vi "Read Voffset.vi"(8 "error in (no error)":errorcluster, 11 "Change Speaker Vparams in":refnum<class "Change Speaker Vparams.lvclass">) -> (0 "error out":errorcluster, 2 "Voffset":dbl, 3 "Change Speaker Vparams out":refnum<class "Change Speaker Vparams.lvclass">)   [LabVIEW 2014, in "ePAS Library.lvlib" / "Change Speaker Vparams.lvclass"]
uses:
  Change Speaker Vparams.lvclass
  Change Speaker Vparams.lvclass/Change Speaker Vparams.ctl
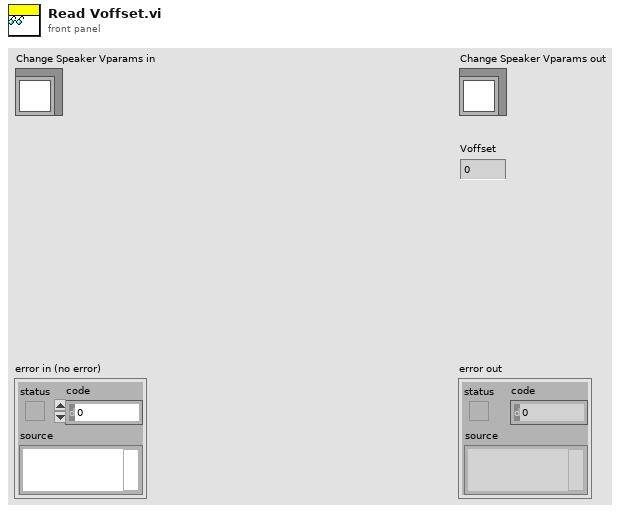
[diagram p1: front panel]
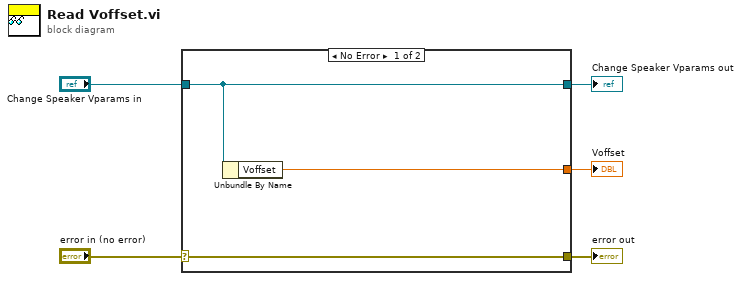
[diagram p0: block diagram]
diagram:
  n1 = case shown="No Error" "error in (no error)" {
    selector: "error in (no error)" -> [w8 w9]
    tunnel: [w8 w9] -> w4
    tunnel: [w7 w10] -> w2
    tunnel: "Change Speaker Vparams in" -> [w7 w10]
    tunnel: [w6 _] -> w1
    frame No Error {
      n2 = Unbundle By Name(w7) -> ("Voffset"=w6:dbl)
    }
    frame Error {
    }
  }
  "error out" <- w4
  "Change Speaker Vparams out" <- w2
  "Voffset" <- w1
